vi "Get Type.vi"(11 "U32 in":refnum<class "U32.lvclass">) -> (3 "Type":string)   [LabVIEW 2017, in "U32.lvclass"]
uses:
  <vilib>/gpm_packages/@cs/data-type-serializer/source/U32/U32.lvclass
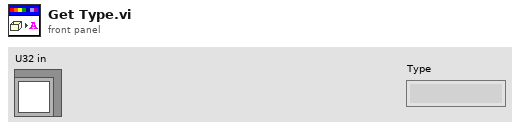
[diagram p1: front panel]
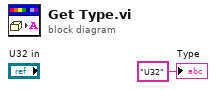
[diagram p0: block diagram]
diagram:
  "Type" <- "U32" ("Type")
